vi "Write Parameter.vi"(8 "error in (no error)":errorcluster, 10 "Parameter":refnum<class "AbstractData.lvclass">, 11 "Set Parameter Msg in":refnum<class "Set Parameter Msg.lvclass">) -> (0 "error out":errorcluster, 3 "Set Parameter Msg out":refnum<class "Set Parameter Msg.lvclass">)   [LabVIEW 2014, in "Set Parameter Msg.lvclass"]
uses:
  Set Parameter Msg.lvclass
  Model/Data/AbstractData/AbstractData.lvclass
  Set Parameter Msg.lvclass/Set Parameter Msg.ctl
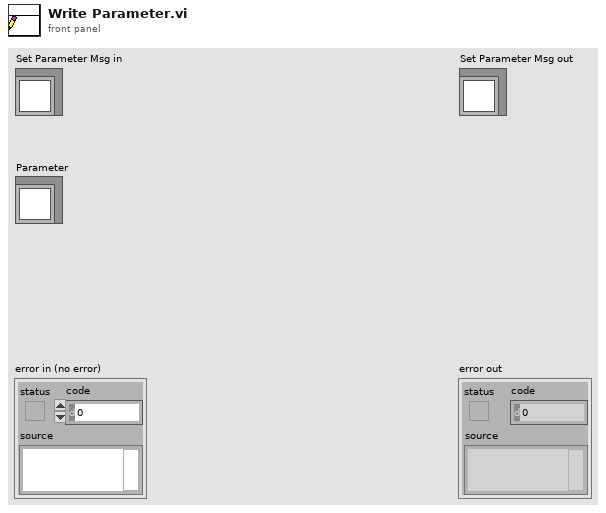
[diagram p1: front panel]
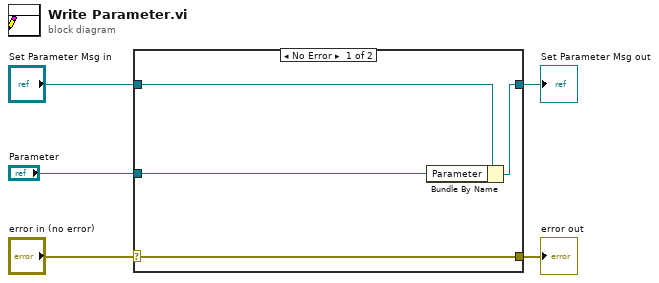
[diagram p0: block diagram]
diagram:
  n1 = case shown="No Error" "error in (no error)" {
    selector: "error in (no error)" -> [w9 w10]
    tunnel: [w9 w10] -> w4
    tunnel: [w7 w11] -> w2
    tunnel: "Set Parameter Msg in" -> [w8 w11]
    tunnel: "Parameter" -> [w6 _]
    frame No Error {
      n2 = Bundle By Name(cluster=w8, "Parameter"=w6) -> (w7:refnum<class "Set Parameter Msg.lvclass">)
    }
    frame Error {
    }
  }
  "error out" <- w4
  "Set Parameter Msg out" <- w2
